vi "UnloadAllBins.vi"(8 "error in (no error)":errorcluster, 11 "JoystickDevRef":T1) -> ()   [LabVIEW 2014]
uses:
  <vilib>/Rock Robotics/WPI/Joystick/WPI_JoystickDevRef.ctl
  <vilib>/Rock Robotics/WPI/Joystick/WPI_JoystickDeviceEnum.ctl
  PlaceTotesEnum.ctl
  Gantry/GantryGlobals.vi
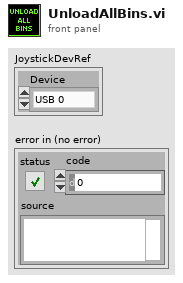
[diagram p1: front panel]
types:
  T1 = typedef "WPI_JoystickDevRef.ctl" = cluster{"Device":T2}
  T2 = typedef "WPI_JoystickDeviceEnum.ctl" = enum16{"USB 0", "USB 1", "USB 2", "USB 3", "USB 4", "USB 5"}
  T3 = typedef "PlaceTotesEnum.ctl" = enum16{"WaitingForInput", "GantryBack", "LiftDown", "LiftUpABit", "GantryOut", "LiftTo0", "GantryTo0"}
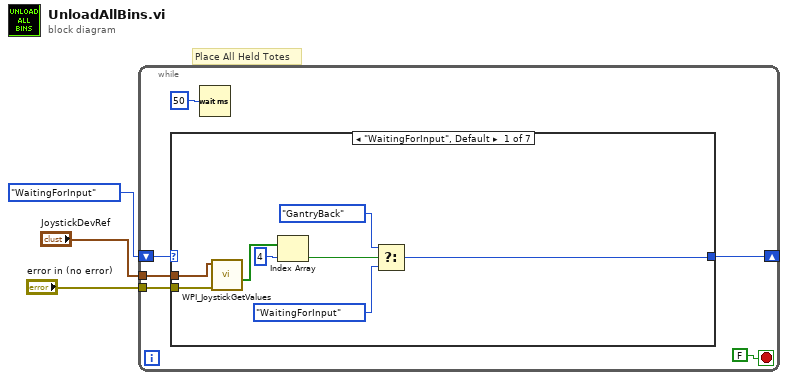
[diagram p0: block diagram]
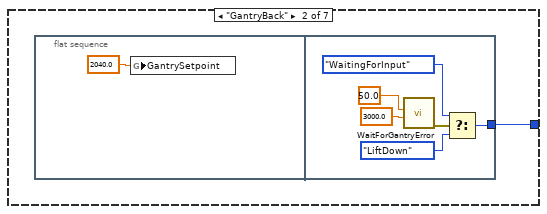
[diagram p2: hidden frame]
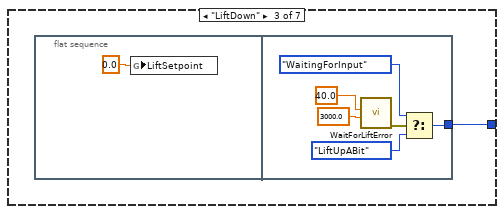
[diagram p3: hidden frame]
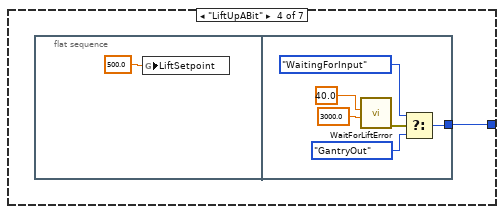
[diagram p4: hidden frame]
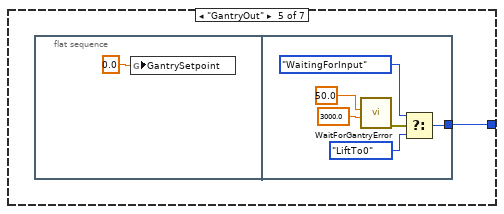
[diagram p5: hidden frame]
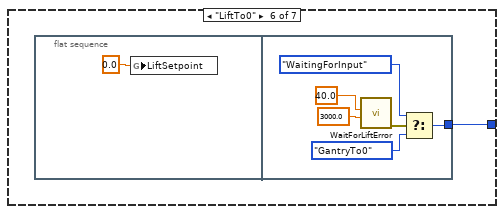
[diagram p6: hidden frame]
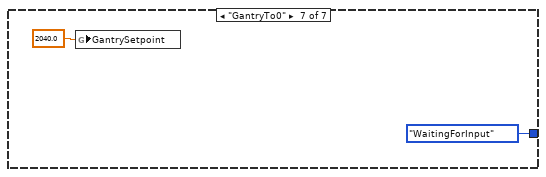
[diagram p7: hidden frame]
diagram:
  # "Place All Held Totes"
  n1 = while {
    shift-right: [w8] -> _
    shift-left: PlaceTotesEnum."WaitingForInput" ("Stuff") -> [w4]
    tunnel: "JoystickDevRef" -> [w6]
    tunnel: "error in (no error)" -> [w5]
    stop <- FALSE stop-if-true
    n2 = case shown="\"WaitingForInput\", Default" w4 {
      tunnel: [w14 w18 w26 w34 w42 w50 PlaceTotesEnum."WaitingForInput" ("Stuff")] -> w8
      tunnel: w6 -> [w11 _ _ _ _ _ _]
      tunnel: w5 -> [w10 _ _ _ _ _ _]
      frame "WaitingForInput", Default {
        n3 = call <vilib>:"WPI_JoystickGetValues.vi"("error in (no error)"=w10, "JoystickDevRef"=w11) -> ("Buttons"=w13:bool[])  [unwired: 5 in, 4 out]
        n4 = Index Array(array=w13, index=4) -> (element=w12:bool)
        n5 = Select(t=PlaceTotesEnum."GantryBack" ("Stuff"), s=w12, f=PlaceTotesEnum."WaitingForInput" ("Stuff")) -> (s? t:f=w14:T3)
      }
      frame "GantryBack" {
        n6 = flat-sequence {
          tunnel: [w23] -> w18
          frame #0 {
            n7 = global write "GantryGlobals.vi" "GantrySetpoint"(2040.0 ("Output")) -> ()
          }
          frame #1 {
            n8 = call "WaitForGantryError.vi"("Timeout (ms)"=3000.0, "AllowedError"=50.0 ("Error")) -> ("error out"=w20:errorcluster)  [unwired: 9 in]
            n9 = Select(t=PlaceTotesEnum."WaitingForInput" ("Stuff"), s=w20, f=PlaceTotesEnum."LiftDown" ("Stuff")) -> (s? t:f=w23:T3)
          }
        }
      }
      frame "LiftDown" {
        n10 = flat-sequence {
          tunnel: [w29] -> w26
          frame #0 {
            n11 = global write "GantryGlobals.vi" "LiftSetpoint"(0.0 ("Output")) -> ()
          }
          frame #1 {
            n12 = call "WaitForLiftError.vi"("Timeout (ms)"=3000.0, "AllowedError"=40.0 ("Error")) -> ("error out"=w28:errorcluster)  [unwired: 9 in]
            n13 = Select(t=PlaceTotesEnum."WaitingForInput" ("Stuff"), s=w28, f=PlaceTotesEnum."LiftUpABit" ("Stuff")) -> (s? t:f=w29:T3)
          }
        }
      }
      frame "LiftUpABit" {
        n14 = flat-sequence {
          tunnel: [w36] -> w34
          frame #0 {
            n15 = global write "GantryGlobals.vi" "LiftSetpoint"(500.0 ("Output")) -> ()
          }
          frame #1 {
            n16 = call "WaitForLiftError.vi"("Timeout (ms)"=3000.0, "AllowedError"=40.0 ("Error")) -> ("error out"=w41:errorcluster)  [unwired: 9 in]
            n17 = Select(t=PlaceTotesEnum."WaitingForInput" ("Stuff"), s=w41, f=PlaceTotesEnum."GantryOut" ("Stuff")) -> (s? t:f=w36:T3)
          }
        }
      }
      frame "GantryOut" {
        n18 = flat-sequence {
          tunnel: [w47] -> w42
          frame #0 {
            n19 = global write "GantryGlobals.vi" "GantrySetpoint"(0.0 ("Output")) -> ()
          }
          frame #1 {
            n20 = call "WaitForGantryError.vi"("Timeout (ms)"=3000.0, "AllowedError"=50.0 ("Error")) -> ("error out"=w44:errorcluster)  [unwired: 9 in]
            n21 = Select(t=PlaceTotesEnum."WaitingForInput" ("Stuff"), s=w44, f=PlaceTotesEnum."LiftTo0" ("Stuff")) -> (s? t:f=w47:T3)
          }
        }
      }
      frame "LiftTo0" {
        n22 = flat-sequence {
          tunnel: [w52] -> w50
          frame #0 {
            n23 = global write "GantryGlobals.vi" "LiftSetpoint"(0.0 ("Output")) -> ()
          }
          frame #1 {
            n24 = call "WaitForLiftError.vi"("Timeout (ms)"=3000.0, "AllowedError"=40.0 ("Error")) -> ("error out"=w57:errorcluster)  [unwired: 9 in]
            n25 = Select(t=PlaceTotesEnum."WaitingForInput" ("Stuff"), s=w57, f=PlaceTotesEnum."GantryTo0" ("Stuff")) -> (s? t:f=w52:T3)
          }
        }
      }
      frame "GantryTo0" {
        n26 = global write "GantryGlobals.vi" "GantrySetpoint"(2040.0 ("Output")) -> ()
      }
    }
    n27 = Wait (ms)(milliseconds to wait=u32 50) -> ()  [unwired: 1 out]
  }
